vi "Reports.Station Configuration Report, Read or Write.vi"(8 "error in (no error)":errorcluster, 9 "Read(F)/Write(T)":bool, 10 "Test Result In":T1={"#attributes"={"Version"="MTE_1.0.0"}, "Station"={"Name"="", "PN"="", "SN"="", "Rev"="", "PC Name"="", "Location"="", "HW_Config"={"HW_Item"=[]}, "SW_Config"={"SW_Item"=[]}}, "Test Run"={"Operator"="", "Start Time"=timestamp(0 s since 1904-01-01), "Duration(s)"=0.0, "Mode"="", "Comment"="", "ProcessStep"=""}, "Test Sequence"={"Name"="", "Config"={"Config_Item"=[]}}, "UUTs"={"UUT"=[]}} {"UUTs"."UUT"."Measurements"."Measurement"."Status" items=["LOG", "PASS", "FAIL", "ERROR"]}, 11 "Config Folder":path) -> (0 "error out":errorcluster, 2 "Test Result Out":T1={"#attributes"={"Version"="MTE_1.0.0"}, "Station"={"Name"="", "PN"="", "SN"="", "Rev"="", "PC Name"="", "Location"="", "HW_Config"={"HW_Item"=[]}, "SW_Config"={"SW_Item"=[]}}, "Test Run"={"Operator"="", "Start Time"=timestamp(0 s since 1904-01-01), "Duration(s)"=0.0, "Mode"="", "Comment"="", "ProcessStep"=""}, "Test Sequence"={"Name"="", "Config"={"Config_Item"=[]}}, "UUTs"={"UUT"=[]}} {"UUTs"."UUT"."Measurements"."Measurement"."Status" items=["LOG", "PASS", "FAIL", "ERROR"]})   [LabVIEW 2024]
uses:
  Report.Result Report File Type.ctl
  Report.Result Report Config.ctl
  <vilib>/KATE/Files/File Utils.lvlib
  Results/Result XML/TestResult.HW Item.ctl
  Results/Result XML/TestResult.SW Item.ctl
  Results/Result XML/TestResult.Station Info.ctl
  Results/Result XML/TestResult.Test Run Info.ctl
  Results/Result XML/TestResult.Test Info.ctl
  Results/Result XML/TestResult.Symptom.State.ctl
  Results/Result XML/TestResult.Symptom.ctl
  Results/Result.Measurement and Attribute Item Status.ctl
  Results/Result XML/TestResult.UUT Result.ctl
  Results/Result XML/TestResult.FullResultData.ctl
  Results/Result.Measurement Item.ctl
  Results/Result XML/TestResult.UUTInfo.ctl
panel:
  out "JSON string":string
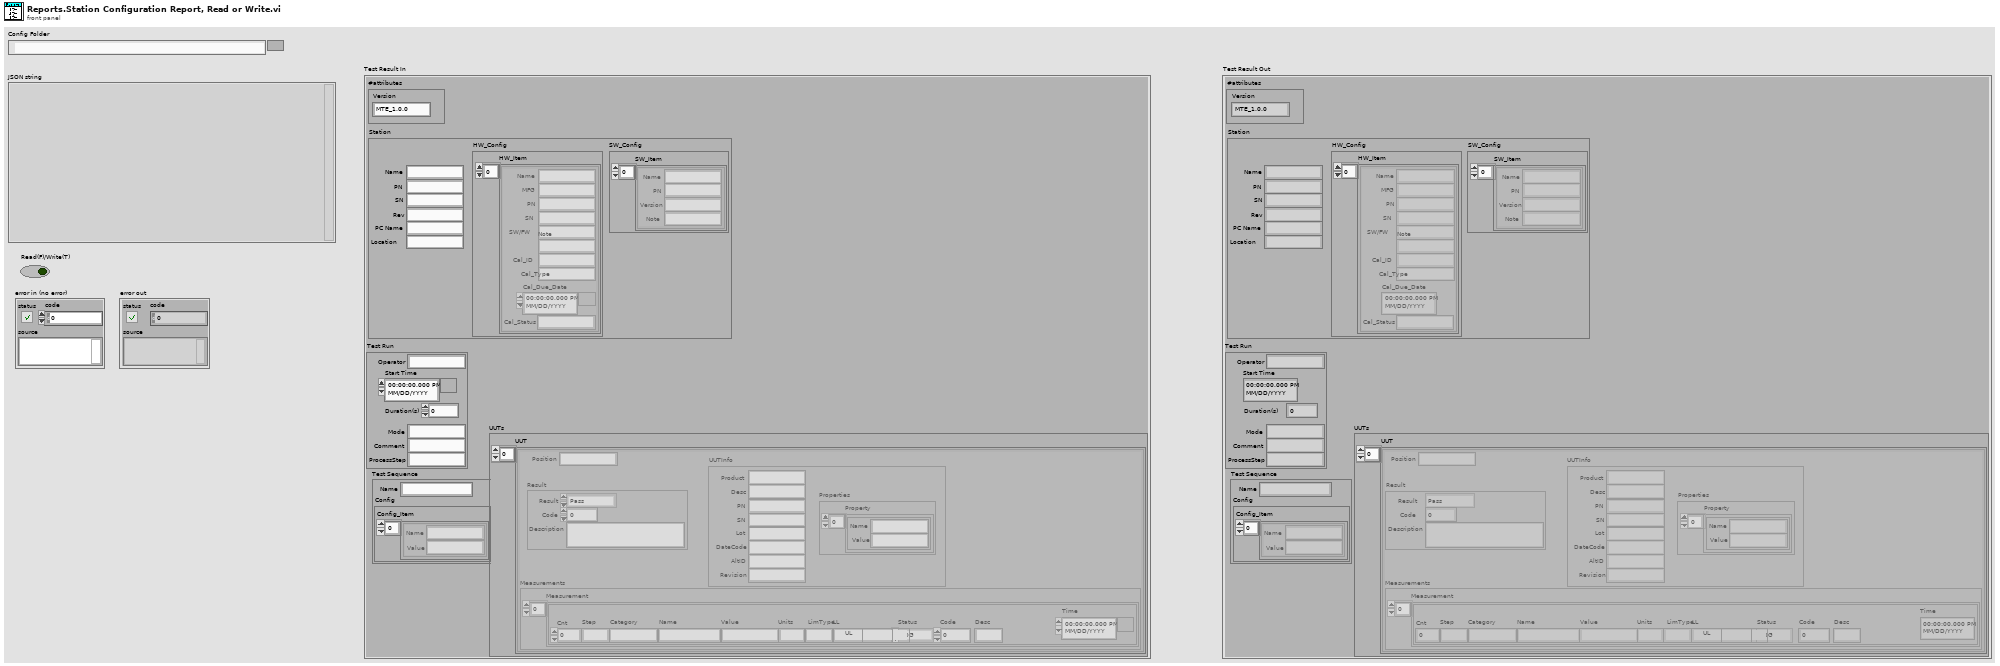
[diagram p1: front panel]
types:
  T1 = typedef "TestResult.FullResultData.ctl" = cluster{"#attributes":cluster{"Version":string}, "Station":T2, "Test Run":T5, "Test Sequence":T6, "UUTs":cluster{"UUT":T7[]}}
  T2 = typedef "TestResult.Station Info.ctl" = cluster{"Name":string, "PN":string, "SN":string, "Rev":string, "PC Name":string, "Location":string, "HW_Config":cluster{"HW_Item":T3[]}, "SW_Config":cluster{"SW_Item":T4[]}}
  T3 = typedef "TestResult.HW Item.ctl" = cluster{"Name":string, "MFG":string, "PN":string, "SN":string, "SW/FW":string, "Note":string, "Cal_ID":string, "Cal_Type":string, "Cal_Due_Date":timestamp, "Cal_Status":string}
  T4 = typedef "TestResult.SW Item.ctl" = cluster{"Name":string, "PN":string, "Version":string, "Note":string}
  T5 = typedef "TestResult.Test Run Info.ctl" = cluster{"Operator":string, "Start Time":timestamp, "Duration(s)":dbl, "Mode":string, "Comment":string, "ProcessStep":string}
  T6 = typedef "TestResult.Test Info.ctl" = cluster{"Name":string, "Config":cluster{"Config_Item":cluster{"Name":string, "Value":string}[]}}
  T7 = typedef "TestResult.UUT Result.ctl" = cluster{"Position":string, "Result":T8, "Measurements":cluster{"Measurement":T10[]}, "UUTInfo":T12}
  T8 = typedef "TestResult.Symptom.ctl" = cluster{"Result":T9, "Code":i32, "Description":string}
  T9 = typedef "TestResult.Symptom.State.ctl" = enum16{"Pass", "Fail", "Error", "Aborted", "Completed", "Logged"}
  T10 = typedef "Result.Measurement Item.ctl" = cluster{"Cnt":i32, "Step":string, "Category":string, "Name":string, "Value":string, "Units":string, "LimType":string, "LL":string, "UL":string, "Status":T11, "Code":i32, "Desc":string, "Time":timestamp}
  T11 = typedef "Result.Measurement and Attribute Item Status.ctl" = i32
  T12 = typedef "TestResult.UUTInfo.ctl" = cluster{"Product":string, "Desc":string, "PN":string, "SN":string, "Lot":string, "DateCode":string, "AltID":string, "Revision":string, "Properties":cluster{"Property":cluster{"Name":string, "Value":string}[]}}
  T13 = typedef "Report.Result Report File Type.ctl" = enum16{"Xlink", "XML_01", "XML_01_wFiles", "JSON_01", "JSON_01_wFiles"}
  T14 = typedef "Report.Result Report Config.ctl" = cluster{"Name":string, "Type":T13, "OutputDir":path}
  T15 = cluster{"Name":string, "Type":string, "Path":string}
  T16 = cluster{"Reports":cluster{"Name":string, "Type":string, "Path":string}[]}
  T17 = cluster{"Name":string, "Type":string, "Path":string}[]
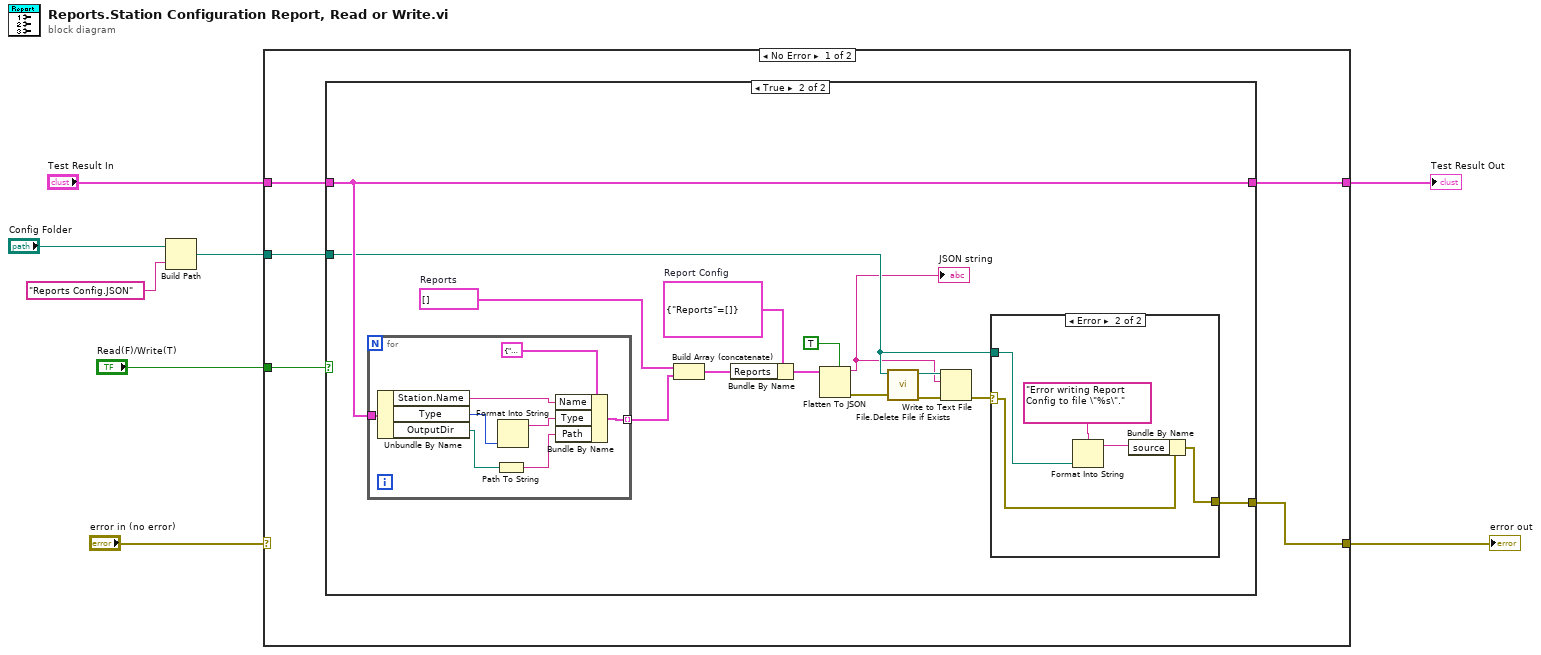
[diagram p0: block diagram]
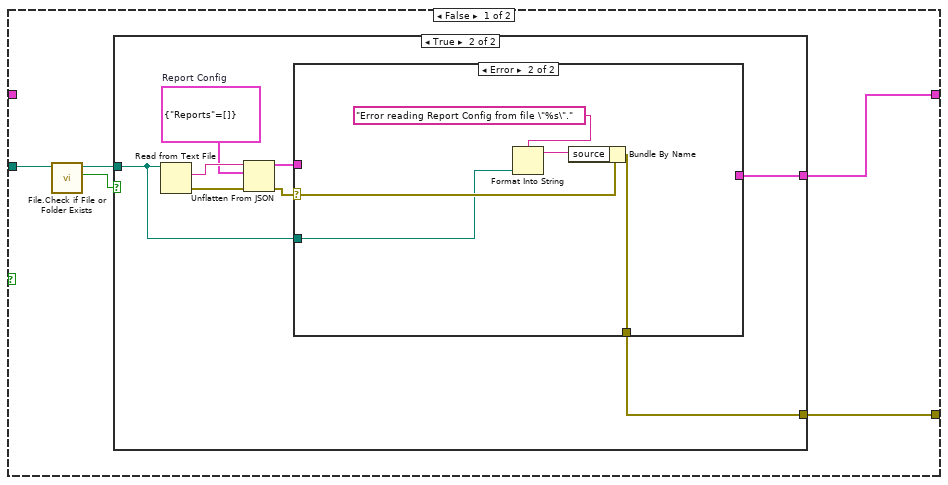
[diagram p2: hidden frame]
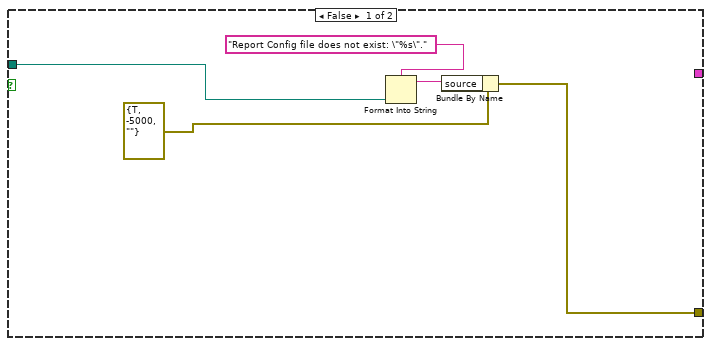
[diagram p3: hidden frame]
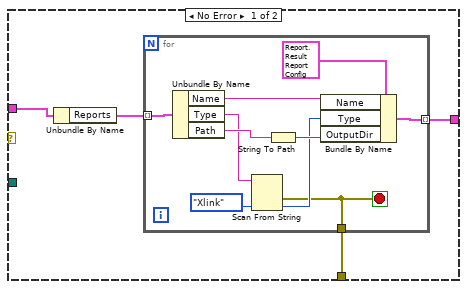
[diagram p4: hidden frame]
diagram:
  n1 = Build Path(base path="Config Folder", name or relative path="Reports Config.JSON") -> (appended path=w2:path)
  n2 = case shown="No Error" "error in (no error)" {
    selector: "error in (no error)" -> [_ w78]
    tunnel: "Read(F)/Write(T)" -> [w13 _]
    tunnel: "Test Result In" -> [w12 w79]
    tunnel: [w9 w79] -> w1
    tunnel: [w10 w78] -> w3
    tunnel: w2 -> [w11 _]
    frame No Error {
      n3 = case shown="True" w13 {
        tunnel: w12 -> [_ w62]
        tunnel: w11 -> [w16 w55]
        tunnel: [w17 w56] -> w10
        tunnel: [w18 w62] -> w9
        frame False {
          n4 = call <vilib>:"File.Check if File or Folder Exists.vi"("Path"=w16) -> ("Exists"=w14:bool, "Dup Path"=w15:path)  [unwired: 6 in, 3 out]
          n5 = case shown="True" w14 {
            tunnel: [_ w29] -> w18
            tunnel: [w19 w28] -> w17
            tunnel: w15 -> [w20 w24]
            frame False {
              n6 = Format Into String(format string="Report Config file does not exist: \"%s\".", w20) -> (resulting string=w23:string)  [unwired: 2 in, 1 out]
              n7 = Bundle By Name(cluster=errorcluster {"status"=TRUE, "code"=-5000, "source"=""} ("error constant"), "source"=w23) -> (w19:errorcluster)
            }
            frame True {
              w25 = T16 {"Reports"=[]}  # Report Config
              n8 = Read from Text File(file (use dialog)=w24) -> (text=w31:string, error out=w26:errorcluster)  [unwired: 3 in, 2 out]
              n9 = Unflatten From JSON(JSON string=w31, type and defaults=w25, error in (no error)=w26) -> (value=w30:T16, error out=w27:errorcluster)  [unwired: 4 in]
              n10 = case shown="Error" w27 {
                selector: w27 -> [_ w50]
                tunnel: w30 -> [w33 _]
                tunnel: [w35 _] -> w29
                tunnel: [w34 w49] -> w28
                tunnel: w24 -> [_ w46]
                frame No Error {
                  n11 = Unbundle By Name(w33) -> ("Reports"=w32:T17)
                  n12 = for {
                    tunnel: w32 -> [w45] mode=indexing
                    tunnel: [w41] -> w35 mode=indexing
                    tunnel: [w36] -> w34
                    stop <- w36 stop-if-true
                    n13 = Unbundle By Name(w45) -> ("Name"=w43:string, "Type"=w39:string, "Path"=w44:string)
                    n14 = Scan From String(input string=w39, default 1=Report.Result_Report_File_Type."Xlink" ("Type")) -> (error out=w36:errorcluster, output 1=w37:T13)  [unwired: 3 in, 2 out]
                    n15 = String To Path(string=w44) -> (path=w42:path)
                    n16 = Bundle By Name(cluster=T14 {"Name"="", "Type"=enum."JSON_01_wFiles", "OutputDir"=path ""} ("Report Config In"), "Name"=w43, "Type"=w37, "OutputDir"=w42) -> (w41:T14)
                  }
                }
                frame Error {
                  n17 = Format Into String(format string="Error reading Report Config from file \"%s\".", w46) -> (resulting string=w48:string)  [unwired: 2 in, 1 out]
                  n18 = Bundle By Name(cluster=w50, "source"=w48) -> (w49:errorcluster)
                }
              }
            }
          }
        }
        frame True {
          w59 = T16 {"Reports"=[]}  # Report Config
          w60 = T17 []  # Reports
          n19 = for {
            tunnel: w62 -> [w77]
            tunnel: [w70] -> w61 mode=indexing
            n20 = Unbundle By Name(w77) -> ("Station.Name"=w73:string, "Type"=w76:T13, "OutputDir"=w75:path)
            n21 = Path To String(path=w75) -> (string=w71:string)
            n22 = Format Into String(w76) -> (resulting string=w72:string)  [unwired: 3 in, 1 out]
            n23 = Bundle By Name(cluster=T15 {"Name"="", "Type"="", "Path"=""} ("Report"), "Name"=w73, "Type"=w72, "Path"=w71) -> (w70:T15)
          }
          n24 = Build Array (concatenate)(w60, w61) -> (w58:T17)
          n25 = Bundle By Name(cluster=w59, "Reports"=w58) -> (w57:T16)
          n26 = Flatten To JSON(enable LabVIEW extensions? (T)=TRUE, anything=w57) -> (JSON string=w51:string, 11:w63:errorcluster)  [unwired: 1 in]
          "JSON string" <- w51
          n27 = call "File.Delete File if Exists.vi"("error in"=w63, "Path"=w55) -> ("error out"=w54:errorcluster, "Path Out"=w53:path)  [unwired: 8 in]
          n28 = Write to Text File(file (use dialog)=w53, text=w51, error in=w54) -> (error out=w52:errorcluster)  [unwired: 1 in, 2 out]
          n29 = case shown="Error" w52 {
            selector: w52 -> [_ w67]
            tunnel: [_ w66] -> w56
            tunnel: w55 -> [_ w65]
            frame No Error {
            }
            frame Error {
              n30 = Format Into String(format string="Error writing Report Config to file \"%s\".", w65) -> (resulting string=w69:string)  [unwired: 2 in, 1 out]
              n31 = Bundle By Name(cluster=w67, "source"=w69) -> (w66:errorcluster)
            }
          }
        }
      }
    }
    frame Error {
    }
  }
  "error out" <- w3
  "Test Result Out" <- w1
